vi "ni579x Configure Clock.vi"(0 "Register Bus":refnum<class "ni579x Register Bus v1 Host.lvclass">=refnum, 1 "scope":string, 5 "clock source":string(combo)="Internal", 7 "reference clock source":string(combo)="Internal", 11 "Error In":errorcluster) -> (4 "Register Bus (out)":refnum<class "ni579x Register Bus v1 Host.lvclass">, 15 "Error Out":errorcluster)   [LabVIEW 2013]
doc: "Configures the source of the sample clock or reference clock.\n\n<B>Input Parameters</B>\n\n<B>Register Bus</B> The Register Bus object created by the ni579x Open VI and used as the session handle for the NI-579x Configuration Design Library.\n\n<B>clock source</B> The source of the Sample Clock. Can be \"Internal\" or the \"ClkIn\" front-panel terminal.\n\n<B>reference clock source</B> The source of the clock that serves as a reference clock for the sample clock and local oscillator. Can be \"Internal\", \"PXI_CLK\" for the PXI backplane reference (sync clock), or \"ClkIn\" for the front-panel terminal.\n\n<B>Output Parameters</B>\n\n<B>Register Bus (out)</B> The Register Bus object created by the ni579x Open VI and used as the session handle for the NI-579x Configuration Design Library."
uses:
  <instrlib>/ni579x/Register Bus/v1/Host/ni579x Register Bus v1 Host.lvclass
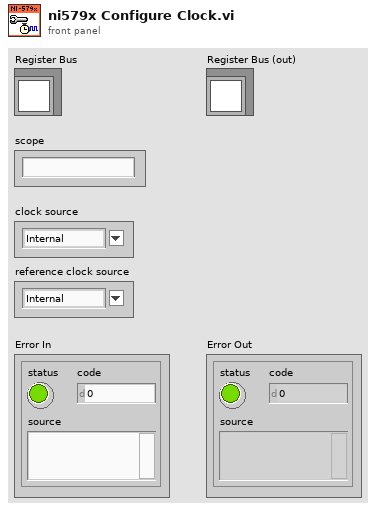
[diagram p1: front panel]
types:
  T1 = typedef "ni579x User Command.ctl" = cluster{"User Data 0":u8, "User Data 1":u8, "User Command ID":T2}
  T2 = typedef "ni579x User Command ID.ctl" = u8
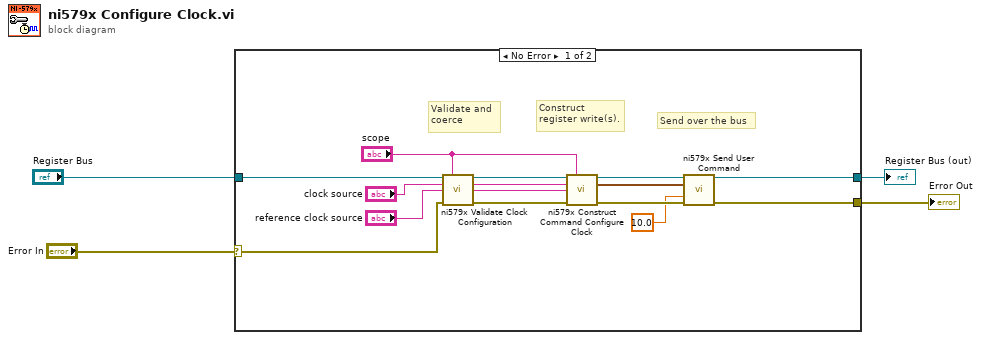
[diagram p0: block diagram]
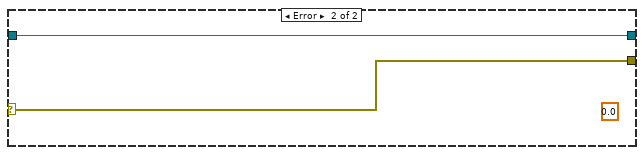
[diagram p2: hidden frame]
diagram:
  n1 = case shown="No Error" "Error In" {
    selector: "Error In" -> [w18 w21]
    tunnel: [w11 w21] -> w3
    tunnel: "Register Bus" -> [w19 w20]
    tunnel: [w12 w20] -> w1
    frame No Error {
      # "Send over the bus"
      # "Construct\nregister write(s)."
      # "Validate and \ncoerce"
      n2 = call <instrlib>:"ni579x Validate Clock Configuration.vi"("Register Bus"=w19, "scope"="scope", "clock source"="clock source", "reference clock source"="reference clock source", "Error In"=w18) -> ("Register Bus (out)"=w16:refnum<class "ni579x Register Bus v1 Host.lvclass">, "coerced clock source"=w8:string, "coerced reference clock source"=w7:string, "Error Out"=w17:errorcluster)  [unwired: 7 in]
      n3 = call <instrlib>:"ni579x Construct Command Configure Clock.vi"("Register Bus"=w16, "scope"="scope", "clock source"=w8, "reference clock source"=w7, "Error In"=w17) -> ("Register Bus (out)"=w14:refnum<class "ni579x Register Bus v1 Host.lvclass">, "User Command"=w6:T1, "Error Out"=w13:errorcluster)  [unwired: 8 in]
      n4 = call <instrlib>:"ni579x Send User Command.vi"("Register Bus"=w14, "User Command"=w6, "timeout"=10.0, "Error In"=w13) -> ("Register Bus (out)"=w12:refnum<class "ni579x Register Bus v1 Host.lvclass">, "Error Out"=w11:errorcluster)  [unwired: 7 in, 3 out]
    }
    frame Error {
      (unwired) 0.0 ("coerced attenuation [dB]")
    }
  }
  "Register Bus (out)" <- w1
  "Error Out" <- w3
